vi "Function Configuration.vi"(4 "Voltage (0: 300 mV)  3":u16(ring)=5 items=["300 mV", "3 V", "30 V", "150/300 V", "3 M Ohms", "10 M Ohms"], 5 "Channel":i8 min=0 max=20 step=1, 6 "Resistance (0: 300 Ohms)  2":u16(ring)=5 items=["300 Ohms", "3 k Ohms", "30 k Ohms", "300 k Ohms", "3 M Ohms", "10 M Ohms"], 7 "Function (5: Temp)":u16(ring)=5 items=["OFF", "VDC", "VAC", "OHMS", "FREQ", "TEMP"], 8 "error in (no error)":errorcluster, 9 "Frequency (0: 900 Hz)":u16(ring)=5 items=["900 Hz", "9 kHz", "90 kHz", "900 kHz", "1 MHz"], 10 "Thermocouple Type (0: J) 2":u16(ring)=5 items=["J", "K", "E", "T", "N", "R", "S", "B", "C"], 11 "VISA resource name":refnum<visa-resource-name>) -> (0 "error out":errorcluster, 1 "read buffer":string, 2 "concatenated string":string, 3 "VISA resource name out":refnum<visa-resource-name>)   [LabVIEW 2010, in "Fluke 2625A.lvlib"]
uses:
  <instrlib>/Fluke 2625A/Fluke 2625A.lvlib
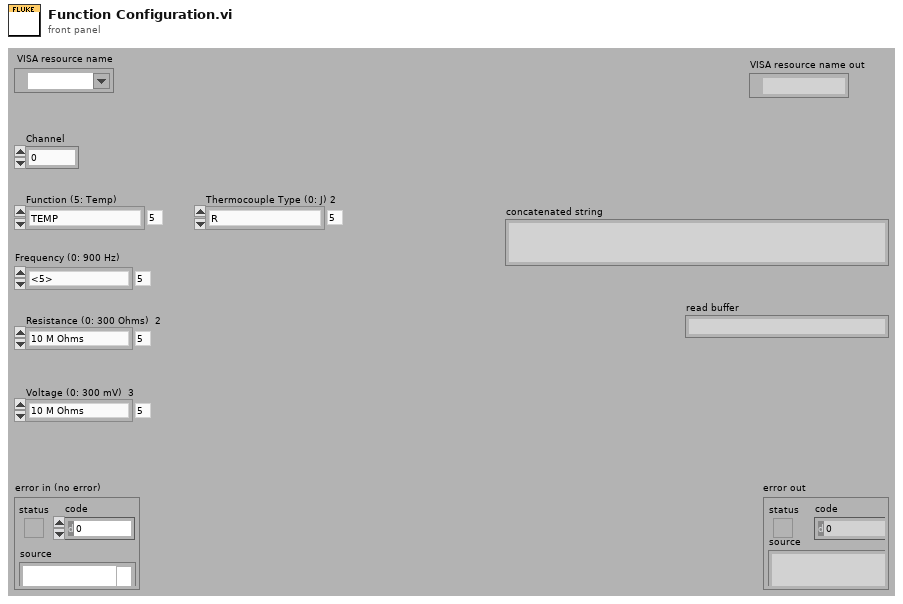
[diagram p1: front panel]
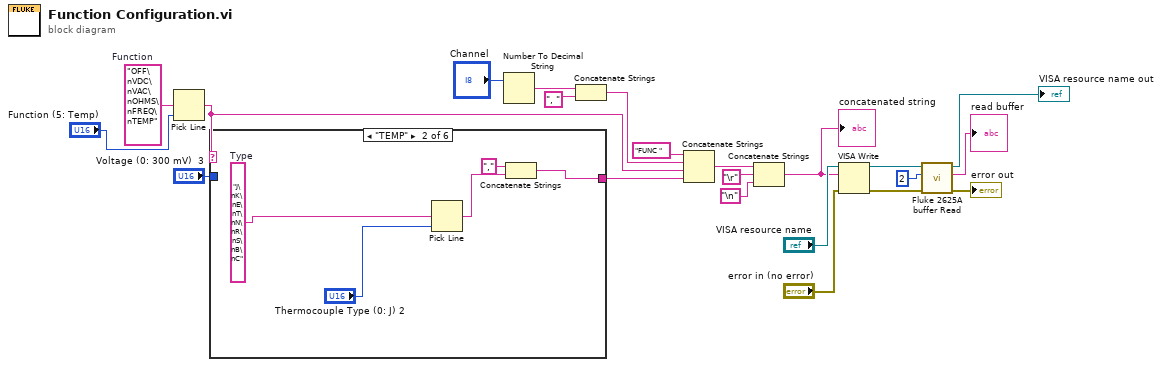
[diagram p0: block diagram]
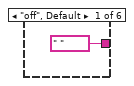
[diagram p2: hidden frame]
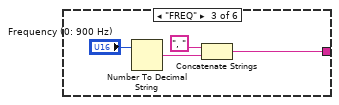
[diagram p3: hidden frame]
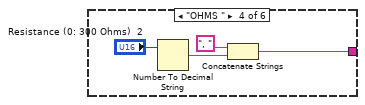
[diagram p4: hidden frame]
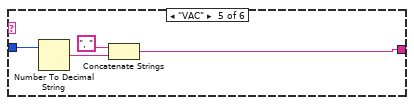
[diagram p5: hidden frame]
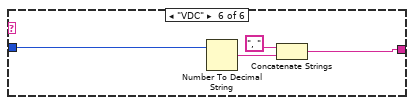
[diagram p6: hidden frame]
diagram:
  w9 = "OFF\nVDC\nVAC\nOHMS\nFREQ\nTEMP"  # Function
  n1 = Pick Line(multi-line string=w9, line index="Function (5: Temp)") -> (output string=w19:string)  [unwired: 1 in]
  n2 = case shown="\"TEMP\"" w19 {
    tunnel: [" " w28 w31 w35 w37 w43] -> w18
    tunnel: "Voltage (0: 300 mV)  3" -> [_ _ _ _ w40 w44]
    frame "off", Default {
    }
    frame "TEMP" {
      w27 = "J\nK\nE\nT\nN\nR\nS\nB\nC"  # Type
      n3 = Pick Line(multi-line string=w27, line index="Thermocouple Type (0: J) 2") -> (output string=w25:string)  [unwired: 1 in]
      n4 = Concatenate Strings("," ("string"), w25) -> (w28:string)
    }
    frame "FREQ" {
      n5 = Number To Decimal String(number="Frequency (0: 900 Hz)") -> (decimal integer string=w29:string)  [unwired: 1 in]
      n6 = Concatenate Strings(", ", w29) -> (w31:string)
    }
    frame "OHMS " {
      n7 = Number To Decimal String(number="Resistance (0: 300 Ohms)  2") -> (decimal integer string=w33:string)  [unwired: 1 in]
      n8 = Concatenate Strings(", ", w33) -> (w35:string)
    }
    frame "VAC" {
      n9 = Number To Decimal String(number=w40) -> (decimal integer string=w38:string)  [unwired: 1 in]
      n10 = Concatenate Strings(", ", w38) -> (w37:string)
    }
    frame "VDC" {
      n11 = Number To Decimal String(number=w44) -> (decimal integer string=w41:string)  [unwired: 1 in]
      n12 = Concatenate Strings(", ", w41) -> (w43:string)
    }
  }
  n13 = Number To Decimal String(number="Channel") -> (decimal integer string=w13:string)  [unwired: 1 in]
  n14 = Concatenate Strings(w13, ", ") -> (w15:string)
  n15 = Concatenate Strings("FUNC ", w15, w19, w18) -> (w16:string)
  n16 = Concatenate Strings(w16, "\r", "\n") -> (w1:string)
  "concatenated string" <- w1
  n17 = VISA Write(VISA resource name="VISA resource name", write buffer=w1, error in (no error)="error in (no error)") -> (VISA resource name out=w4:refnum<visa-resource-name>, error out=w5:errorcluster)  [unwired: 1 out]
  n18 = call <instrlib>:"Fluke 2625A buffer Read.vi"("error out"=w5, "byte count"=u32 2, "VISA resource name out"=w4) -> ("error out 2"=→"error out":errorcluster, "read buffer"=→"read buffer":string, "VISA resource name out 2"=→"VISA resource name out":refnum<visa-resource-name>)  [unwired: 6 in]
